vi "viUpdate.vi"(8 "error in (no error)":errorcluster, 11 "OutputPath":path) -> (0 "error out":errorcluster)   [LabVIEW 2016]
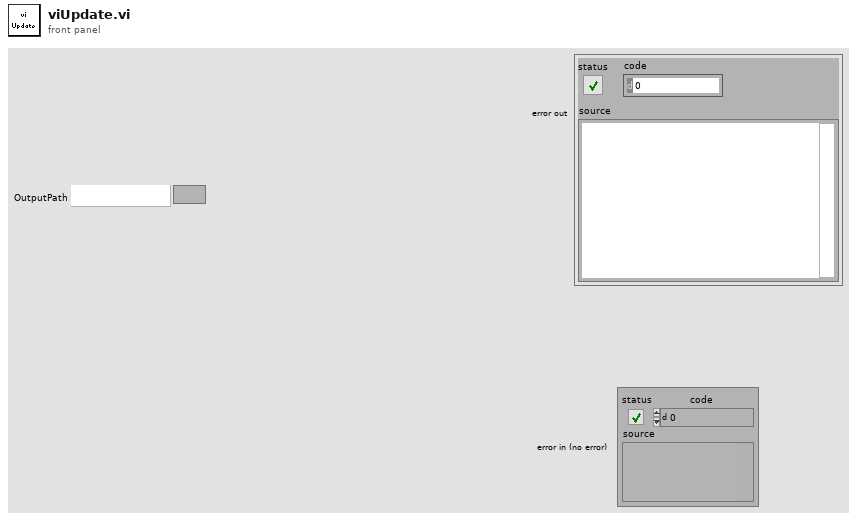
[diagram p1: front panel]
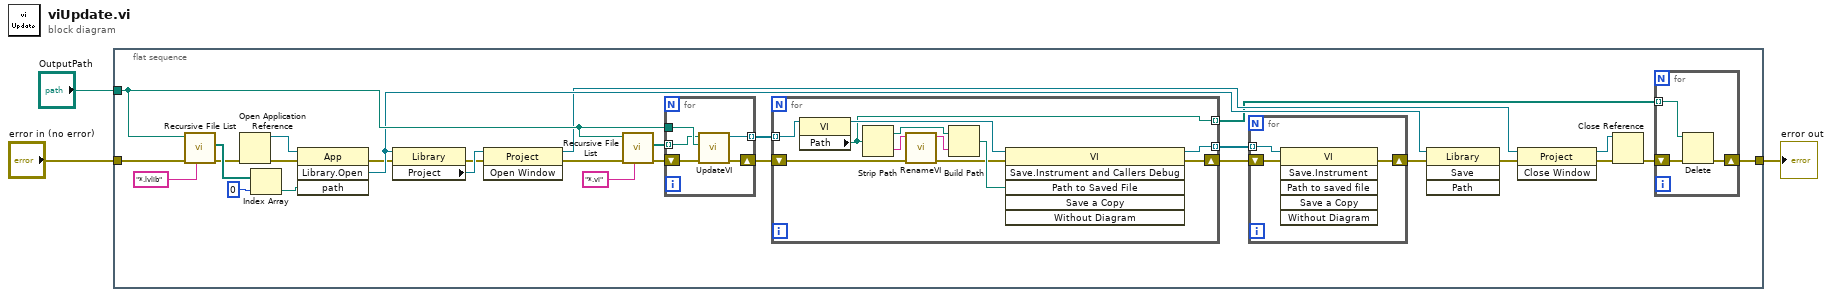
[diagram p0: block diagram]
diagram:
  n1 = flat-sequence {
    tunnel: "OutputPath" -> [w29]
    tunnel: [w5] -> w2
    tunnel: "error in (no error)" -> [w24]
    frame #0 {
      n2 = call <vilib>:"Recursive File List.vi"("pattern"="*.lvlib", "error in (no error)"=w24, "Folder Path"=w29) -> ("error out"=w25:errorcluster, "All Files in Dir"=w27:path[])  [unwired: 4 in, 3 out]
      n3 = Open Application Reference(8:w25) -> (0:w22:errorcluster, 3:w23:refnum<vi>)  [unwired: 3 in]
      n4 = Index Array(array=w27, index=0) -> (element=w21:path)
      n5 = invoke class="App" method="Library.Open"(reference=w23, error in=w22, "path"=w21) -> (error out=w13:errorcluster, "Open Library"=w15:refnum<vi>)  [unwired: 1 in, 2 out]
      n6 = property class="Library"(reference=w15, error in=w13) -> (error out=w12:errorcluster, "Project"=w14:refnum<vi>)  [unwired: 1 out]
      n7 = invoke class="Project" method="Open Window"(reference=w14, error in=w12) -> (reference out=w10:refnum<vi>, error out=w11:errorcluster)  [unwired: 1 in, 1 out]
      n8 = call <vilib>:"Recursive File List.vi"("pattern"="*.vi", "error in (no error)"=w11, "Folder Path"=w29) -> ("error out"=w30:errorcluster, "All Files in Dir"=w31:path[])  [unwired: 4 in, 3 out]
      n9 = for {
        tunnel: w31 -> [w37] mode=indexing
        tunnel: w29 -> [w40]
        shift-right: [w38] -> w16
        shift-left: w30 -> [w39]
        tunnel: [w36] -> w17 mode=indexing
        n10 = call "UpdateVI.vi"("error in (no error)"=w39, "Controls"=w40, "VIToUpdate"=w37) -> ("error out"=w38:errorcluster, "reference out"=w36:refnum<vi>)  [unwired: 7 in]
      }
      n11 = for {
        shift-right: [w54] -> w20
        shift-left: w16 -> [w48]
        tunnel: w17 -> [w46] mode=indexing
        tunnel: [w47] -> w19 mode=indexing
        tunnel: [w44] -> w4 mode=indexing
        n12 = property class="VI"(reference=w46) -> (reference out=w45:refnum<vi>, "Path"=w44:path)  [unwired: 1 in, 1 out]
        n13 = Strip Path(path=w44) -> (stripped path=w51:path, name=w53:string)
        n14 = call "RenameVI.vi"("error in (no error)"=w48, "InitialName"=w53) -> ("error out"=w49:errorcluster, "NewName"=w52:string)  [unwired: 8 in]
        n15 = Build Path(base path=w51, name or relative path=w52) -> (appended path=w50:path)
        n16 = invoke class="VI" method="Save.Instrument and Callers Debug"(reference=w45, error in=w49, "Path to Saved File"=w50) -> (reference out=w47:refnum<vi>, error out=w54:errorcluster)  [unwired: 3 in, 4 out]
      }
      n17 = for {
        shift-right: [w42] -> w18
        shift-left: w20 -> [w43]
        tunnel: w19 -> [w41] mode=indexing
        n18 = invoke class="VI" method="Save.Instrument"(reference=w41, error in=w43) -> (error out=w42:errorcluster)  [unwired: 4 in, 5 out]
      }
      n19 = invoke class="Library" method="Save"(reference=w15, error in=w18) -> (error out=w9:errorcluster)  [unwired: 2 in, 3 out]
      n20 = invoke class="Project" method="Close Window"(reference=w10, error in=w9) -> (reference out=w7:refnum<vi>, error out=w8:errorcluster)  [unwired: 1 in, 1 out]
      n21 = Close Reference(reference=w7, error in (no error)=w8) -> (error out=w6:errorcluster)
      n22 = for {
        shift-right: [w34] -> w5
        shift-left: w6 -> [w35]
        tunnel: w4 -> [w33] mode=indexing
        n23 = Delete(path (use dialog)=w33, error in=w35) -> (error out=w34:errorcluster)  [unwired: 3 in, 2 out]
      }
    }
  }
  "error out" <- w2
